vi "removeEdge.vi"(0 "reference":refnum<class "CallNode.lvclass">, 1 "graph":refnum<class "Graph.lvclass">, 2 "edge":refnum<class "AbstractEdge.lvclass">, 5 "error in (no error)":errorcluster) -> (14 "reference out":refnum<class "CallNode.lvclass">, 19 "error out":errorcluster)   [LabVIEW 2016, in "CallNode.lvclass"]
uses:
  <resource>/Framework/Providers/Open_GDS/UML/CallNode_class/CallNode.lvclass
  C:/Program Files (x86)/National Instruments/LabVIEW 2016/resource/Framework/Providers/Open_GDS/UML/AbstractNode_class/AbstractNode.lvclass
  <resource>/Framework/Providers/Open_GDS/UML/Graph_class/Graph.lvclass
  <resource>/Framework/Providers/Open_GDS/UML/AbstractEdge_class/AbstractEdge.lvclass
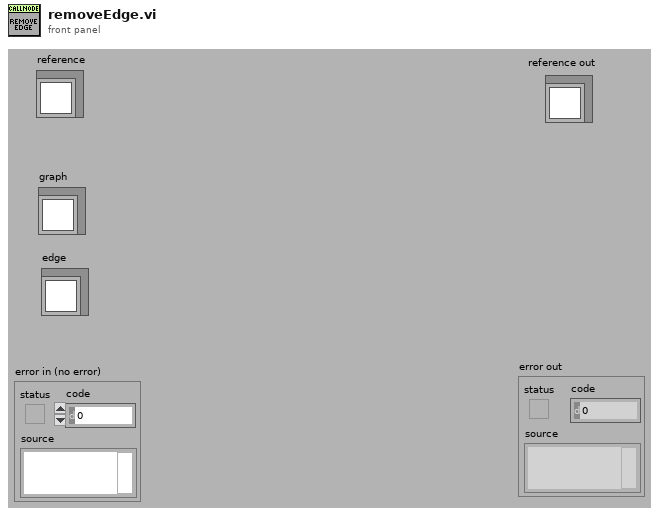
[diagram p1: front panel]
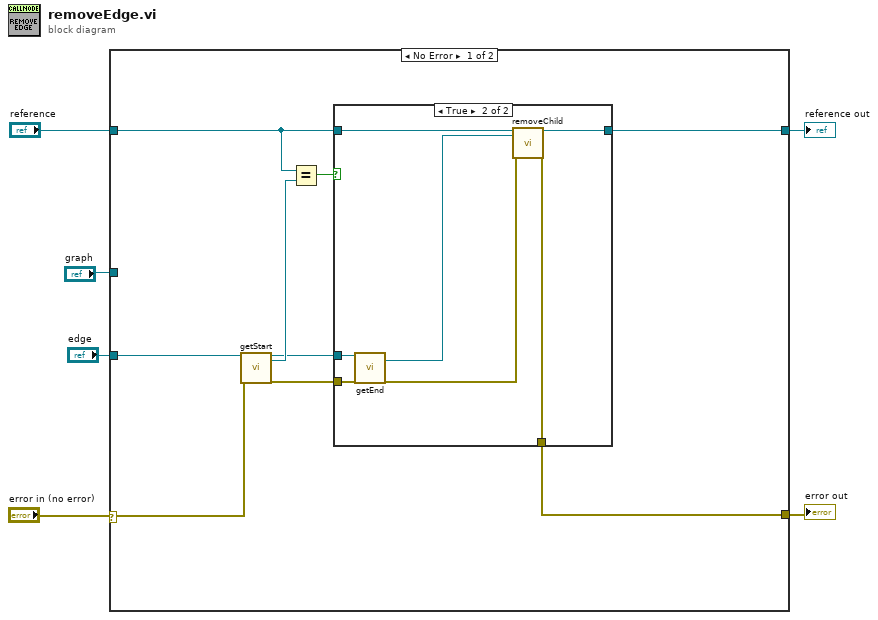
[diagram p0: block diagram]
diagram:
  n1 = case shown="No Error" "error in (no error)" {
    selector: "error in (no error)" -> [w12 w25]
    tunnel: "reference" -> [w15 w26]
    tunnel: [w14 w25] -> w5
    tunnel: [w13 w26] -> w4
    tunnel: "graph" -> [_ _]
    tunnel: "edge" -> [w11 _]
    frame No Error {
      n2 = call-dynamic "getStart.vi"("reference"=w11, "error in (no error)"=w12) -> ("reference out"=w7:refnum<class "AbstractEdge.lvclass">, "startNode"=w10:refnum<class "AbstractNode.lvclass">, "error out"=w8:errorcluster)  [unwired: 14 in, 1 out]
      n3 = Equal?(x=w15, y=w10) -> (x = y?=w9:bool)
      n4 = case shown="True" w9 {
        tunnel: [w16 w24] -> w13
        tunnel: [w17 w23] -> w14
        tunnel: w15 -> [w16 w22]
        tunnel: w8 -> [w17 w21]
        tunnel: w7 -> [_ w20]
        frame False {
        }
        frame True {
          n5 = call-dynamic "getEnd.vi"("reference"=w20, "error in (no error)"=w21) -> ("endNode"=w19:refnum<class "AbstractNode.lvclass">, "error out"=w18:errorcluster)  [unwired: 14 in, 2 out]
          n6 = call-dynamic "removeChild.vi"("reference"=w22, "node"=w19, "error in (no error)"=w18) -> ("reference out"=w24:refnum<class "CallNode.lvclass">, "error out"=w23:errorcluster)  [unwired: 15 in]
        }
      }
    }
    frame Error {
    }
  }
  "reference out" <- w4
  "error out" <- w5
